vi "난수일치.vi"() -> ()   [LabVIEW 2014]
panel:
  out "x+1":i32
  out "숫자형 2":dbl
  in  "숫자형":dbl min=0.0 max=1000.0 step=1.0
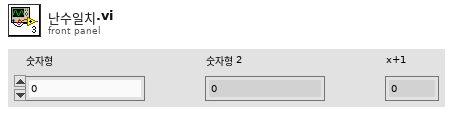
[diagram p1: front panel]
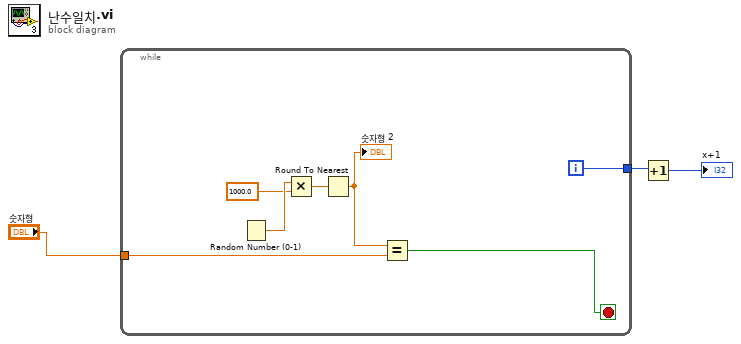
[diagram p0: block diagram]
diagram:
  n1 = while {
    tunnel: "숫자형" -> [w6]
    tunnel: [w4] -> w2
    i -> [w4]
    stop <- w5 stop-if-true
    n2 = Random Number (0-1)() -> (number: 0 to 1=w10:dbl)
    n3 = Multiply(x=w10, y=1000.0) -> (x*y=w8:dbl)
    n4 = Round To Nearest(number=w8) -> (nearest integer value=w7:dbl)
    "숫자형 2" <- w7
    n5 = Equal?(x=w7, y=w6) -> (x = y?=w5:bool)
  }
  n6 = Increment(x=w2) -> (x+1=→"x+1":i32)
